vi "DependencyChecker_Example.vi"() -> ()   [LabVIEW 2020]
uses:
  DependencyChecker/LibraryDependentInfo.vi
  <vilib>/Utility/lvfile.llb/FT_FileTypes.ctl
  DependencyChecker/FilterOptions.ctl
  DependencyChecker/DependencyChecker.lvlib
  VISJS-Viewer/VISJS Viewer.lvlib
  <vilib>/Utility/lvfile.llb/NI_FileType.lvlib
panel:
  out "LibraryDependencies":map{path, T1}(c390)
  in  "File Path":path=path "C:/Projects/DesignPatterns/Decorator1"
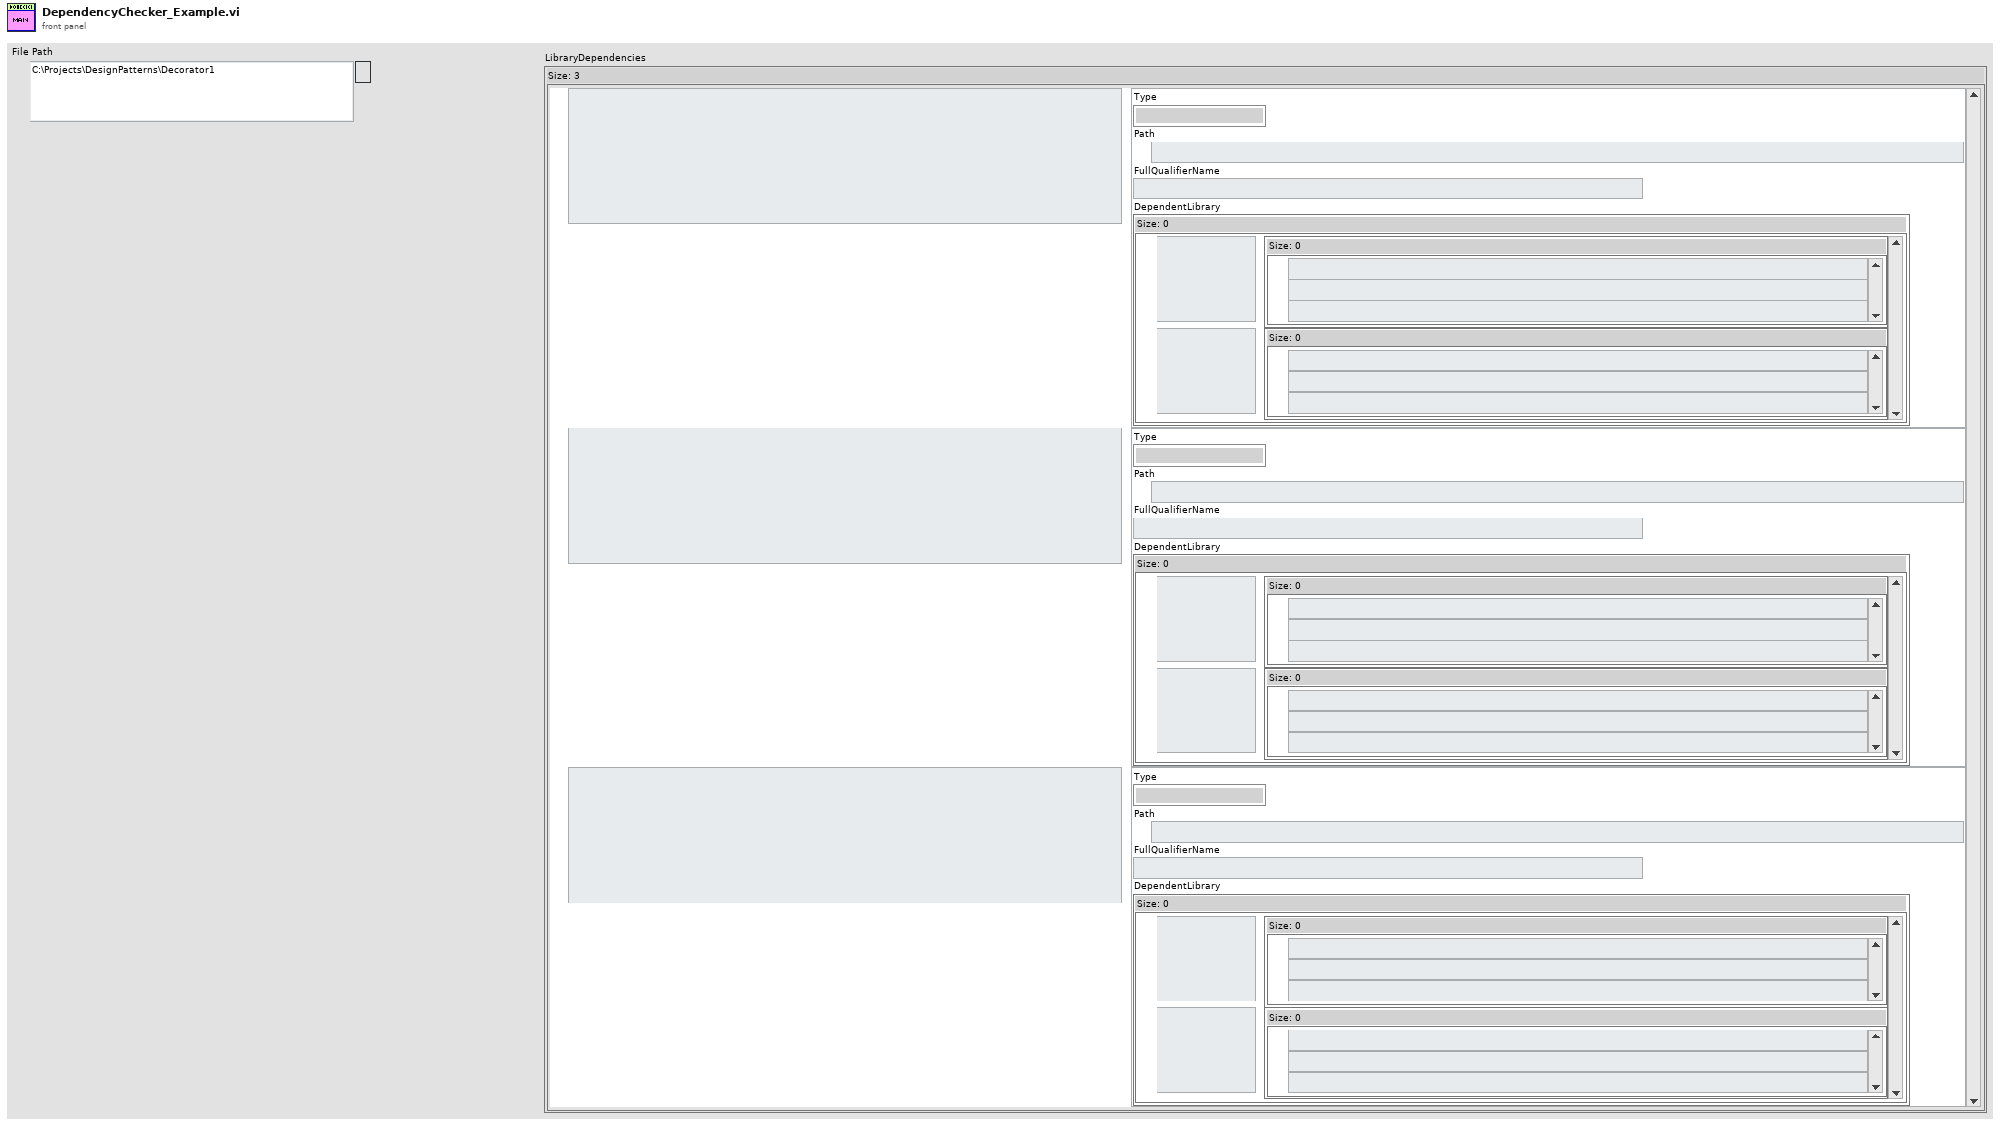
[diagram p1: front panel]
types:
  T1 = typedef "DependencyChecker.lvlib/LibraryDependentInfo.vi" = cluster{"Type":T2, "Path":path, "FullQualifierName":string, "DependentLibrary":map{path, set{path}}}
  T2 = typedef "NI_FileType.lvlib/FT_FileTypes.ctl" = enum32{"Invalid file/path", "Unknown type", "Instrument", "Control", "Polymorphic VI", "Project", "Library", "LVClass", "XControl", "XNode", "CIN", "Run-time menu", "Palette menu", "LLB", "Shortcut", "Directory", "Class Private Data Control", "Statechart", "MathScript .m file", "Ladder Diagram", "LVLibp"}
  T3 = typedef "DependencyChecker.lvlib/FilterOptions.ctl" = cluster{"Ignore user.lib":bool, "Ignore vi.lib":bool, "Ignore instr.lib":bool, "FolderToIgnore":path[], "Ignore libraries":bool, "Ignore lvcasses":bool, "Ignore xnodes":bool, "Ignore xcontrols":bool, "Ignore Channel Classes":bool}
  T4 = enum16{"All Classes and Libraries", "Libraries and Classes not belonging to any library", "Only Classes", "Only Libraries", "Only Libraries (no sub libraries)", "Only Items with Circular Dependencies"}
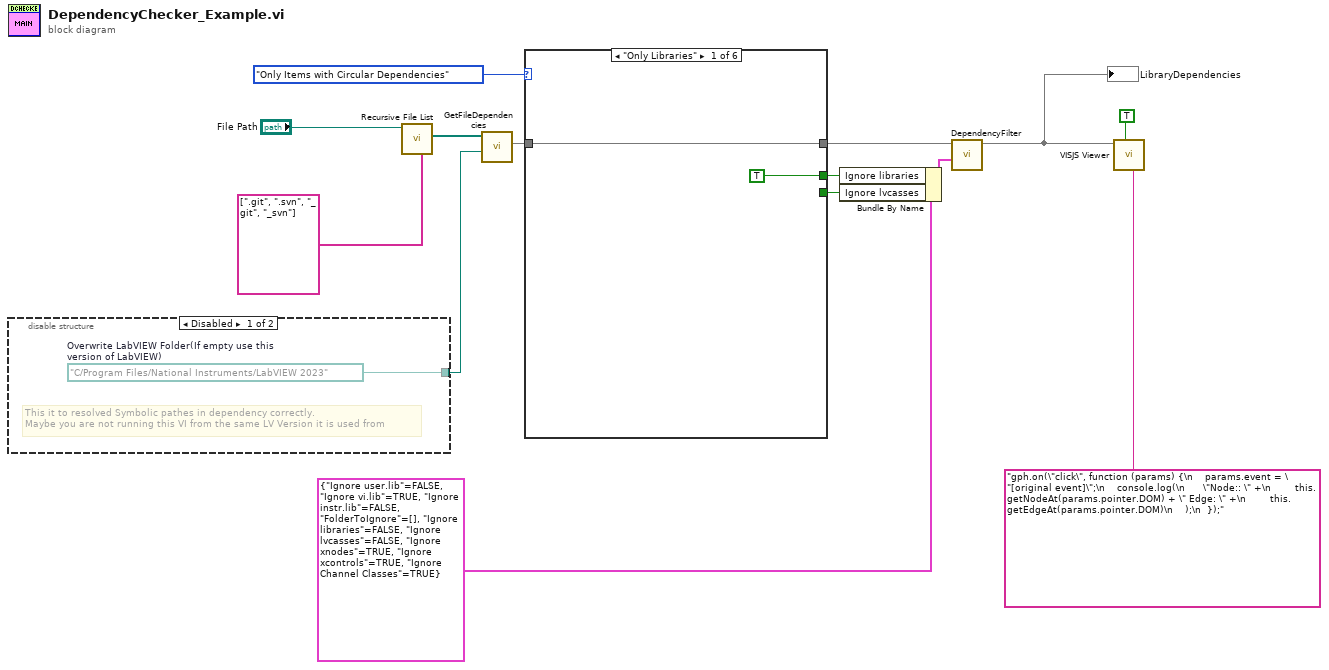
[diagram p0: block diagram]
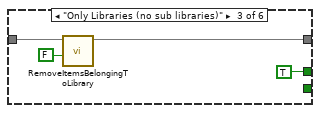
[diagram p3: hidden frame]
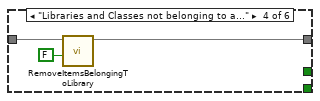
[diagram p4: hidden frame]
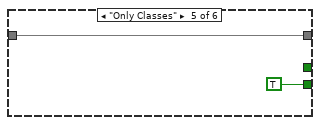
[diagram p5: hidden frame]
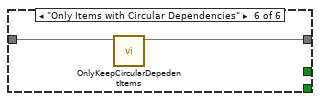
[diagram p6: hidden frame]
diagram:
  n1 = disable-structure shown="Disabled" {
    disable-tunnel: [w15 _] -> w10
    frame Disabled {
      w15 = path "C:/Program Files/National Instruments/LabVIEW 2023"  # Overwrite LabVIEW Folder(If empty use this version of LabVIEW)
      # "This it to resolved Symbolic pathes in dependency correctly.\nMaybe you are not running this VI from the same LV Version it is used from"
    }
    frame Enabled {
    }
  }
  n2 = call <vilib>:"Recursive File List.vi"("Folders to Exclude"=string[] [".git", ".svn", "_git", "_svn"], "Folder Path"="File Path") -> ("All Files in Dir"=w13:path[])  [unwired: 5 in, 4 out]
  n3 = call "GetFileDependencies.vi"("Overwrite LabVIEW Folder(If empty use this version of LabVIEW)"=w10, "All Files in Dir"=w13) -> ("LibraryDependency"=w8:map{path, T1})  [unwired: 8 in, 1 out]
  n4 = case shown="\"Only Libraries\"" T4."Only Items with Circular Dependencies" {
    tunnel: [w17 w18 w20 w23 w26 w28] -> w6
    tunnel: w8 -> [w17 w18 w22 w25 w26 w29]
    tunnel: [TRUE _ TRUE _ _ _] -> w2
    tunnel: [_ _ _ _ TRUE _] -> w1
    frame "Only Libraries" {
    }
    frame "All Classes and Libraries" {
    }
    frame "Only Libraries (no sub libraries)" {
      n5 = call "RemoveItemsBelongingToLibrary.vi"("EvenSubLibraries"=FALSE, "LibraryDependency In"=w22) -> ("LibraryDependency Out"=w20:map{path, T1})  [unwired: 9 in]
    }
    frame "Libraries and Classes not belonging to any library" {
      n6 = call "RemoveItemsBelongingToLibrary.vi"("EvenSubLibraries"=FALSE, "LibraryDependency In"=w25) -> ("LibraryDependency Out"=w23:map{path, T1})  [unwired: 9 in]
    }
    frame "Only Classes" {
    }
    frame "Only Items with Circular Dependencies" {
      n7 = call "OnlyKeepCircularDepedentItems.vi"("LibraryDependency In"=w29) -> ("LibraryDependency Out"=w28:map{path, T1})  [unwired: 10 in]
    }
  }
  n8 = Bundle By Name(cluster=T3 {"Ignore user.lib"=FALSE, "Ignore vi.lib"=TRUE, "Ignore instr.lib"=FALSE, "FolderToIgnore"=[], "Ignore libraries"=FALSE, "Ignore lvcasses"=FALSE, "Ignore xnodes"=TRUE, "Ignore xcontrols"=TRUE, "Ignore Channel Classes"=TRUE} ("FilterOptions"), "Ignore libraries"=w2, "Ignore lvcasses"=w1) -> (w4:T3)
  n9 = call "DependencyFilter.vi"("FilterOptions"=w4, "LibraryDependency In"=w6) -> ("Filtered LibraryDependency Out"=w5:map{path, T1})  [unwired: 9 in]
  "LibraryDependencies" <- w5
  n10 = call "VISJS Viewer.vi"("Extra Scripts"="gph.on(\"click\", function (params) {\n    params.event = \"[original event]\";\n    console.log(\n      \"Node:: \" +\n        this.getNodeAt(params.pointer.DOM) + \" Edge: \" +\n        this.getEdgeAt(params.pointer.DOM)\n    );\n  });" ("Options"), "OpenWebBrowser(False)"=TRUE, "LibraryDependency"=w5) -> ()  [unwired: 7 in, 2 out]
